vi "生成sin函数.vi"() -> ()   [LabVIEW 2019]
panel:
  out "x/y":sgl
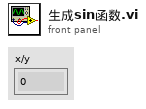
[diagram p1: front panel]
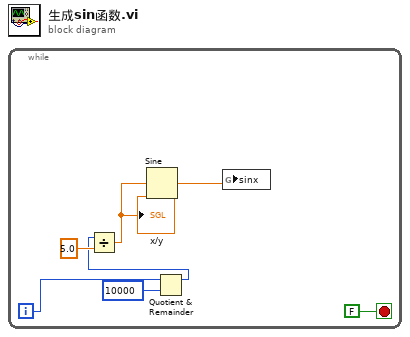
[diagram p0: block diagram]
diagram:
  n1 = while {
    i -> [w3]
    stop <- FALSE stop-if-true
    n2 = Quotient & Remainder(x=w3, y=10000) -> (x-y*floor(x/y)=w1:i32)  [unwired: 1 out]
    n3 = Divide(x=w1, y=sgl 5.0) -> (x/y=w5:sgl)
    "x/y" <- w5
    n4 = Sine(x=w5) -> (sin(x)=w6:sgl)
    n5 = global write "sinx.vi" "sinx"(w6) -> ()
  }
